vi "Out_S1F13.vi"(7 "Host":bool, 8 "error in (no error)":errorcluster, 10 "S1F13":T1, 11 "S1 Message Class in":refnum<class "S1 Message Class.lvclass">) -> (0 "error out":errorcluster, 3 "S1 Message Class out":refnum<class "S1 Message Class.lvclass">)   [LabVIEW 2020, in "SECS Communication.lvlib" / "S1 Message Class.lvclass"]
uses:
  S1 Message Class.lvclass
  D:/Dropbox/SECS/LabVIEW Code/Com/SECS Communication/SECS-II Class/SECS-II Class.lvclass
  S1F13.ctl
  SECS-II Class/Data Message_List.vi
  SECS-II Class/Data Message_ASCII.vi
  S1 Message Class.lvclass/S1 Message Class.ctl
  SECS-II Class/SECS-II Class.lvclass
  D:/Dropbox/SECS/LabVIEW Code/Com/SECS Communication/S1 Message Class/S1 Message Class.lvclass
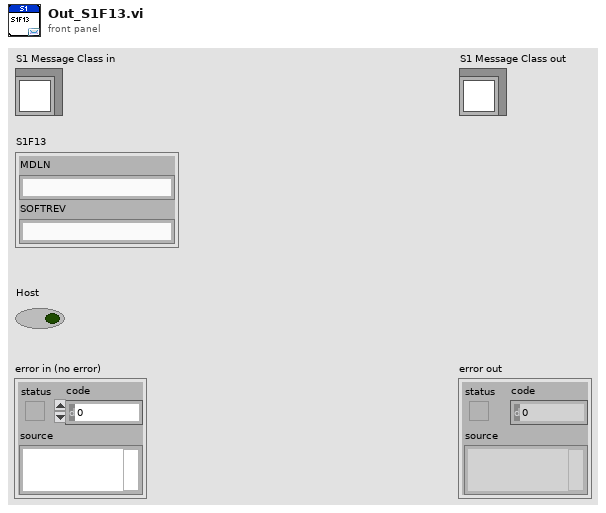
[diagram p1: front panel]
types:
  T1 = typedef "SECS Communication.lvlib/S1 Message Class.lvclass/S1F13.ctl" = cluster{"MDLN":string, "SOFTREV":string}
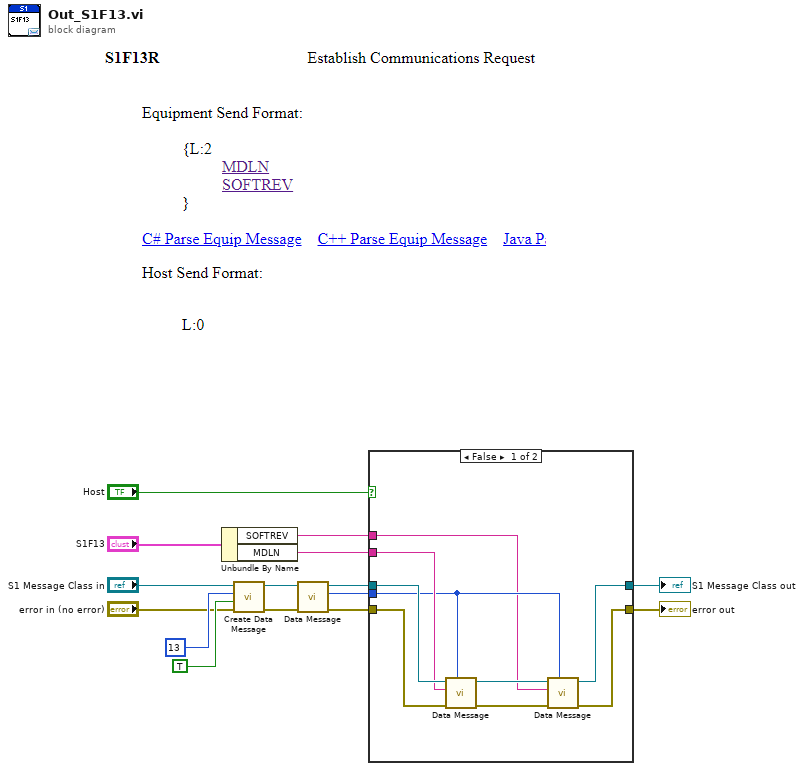
[diagram p0: block diagram]
diagram:
  n1 = Unbundle By Name("S1F13") -> ("SOFTREV"=w2:string, "MDLN"=w1:string)
  n2 = call "Create Data Message.vi"("error in (no error)"="error in (no error)", "W-Bit"=TRUE, "Function"=u8 13, "SECS-II Class in"="S1 Message Class in") -> ("error out"=w10:errorcluster, "SECS-II Class out"=w11:refnum<class "S1 Message Class.lvclass">)  [unwired: 6 in]
  n3 = call-poly "Data Message.vi"("error in"=w10, "SECS-II Class in"=w11) -> ("error out"=w9:errorcluster, "Index"=w7:i32, "SECS-II Class out"=w8:refnum<class "S1 Message Class.lvclass">)  [unwired: 7 in]
  n4 = case shown="False" "Host" {
    tunnel: w9 -> [w24 w26]
    tunnel: w8 -> [w23 w25]
    tunnel: w1 -> [w22 _]
    tunnel: w7 -> [w19 _]
    tunnel: w2 -> [w18 _]
    tunnel: [w17 w26] -> w6
    tunnel: [w16 w25] -> w5
    frame False {
      n5 = call-poly "Data Message.vi"("Parent Index"=w19, "error in"=w24, "Data"=w22, "SECS-II Class in"=w23) -> ("error out"=w20:errorcluster, "SECS-II Class out"=w21:refnum<class "S1 Message Class.lvclass">)  [unwired: 6 in]
      n6 = call-poly "Data Message.vi"("Parent Index"=w19, "error in"=w20, "Data"=w18, "SECS-II Class in"=w21) -> ("error out"=w17:errorcluster, "SECS-II Class out"=w16:refnum<class "S1 Message Class.lvclass">)  [unwired: 6 in]
    }
    frame True {
    }
  }
  "error out" <- w6
  "S1 Message Class out" <- w5
